vi "Database.Main-Select.vi"(8 "error in":errorcluster, 10 "Values":T1 {"Values" format="%.3f"}) -> (0 "error out":errorcluster, 2 "Saved":bool)   [LabVIEW 2016]
doc: "Go to DB->WriteStationValues action\nReturn boolean flag to show if data was saved to DB successfully\n\nWabco 2017 All right reserved\nAuthor: maciej.szupienko@wabco-auto.com"
uses:
  Database.Main.Data.PrevStation.ctl
  Sequence/Sequence.Step.Status.ctl
  Database.Main.Action.ctl
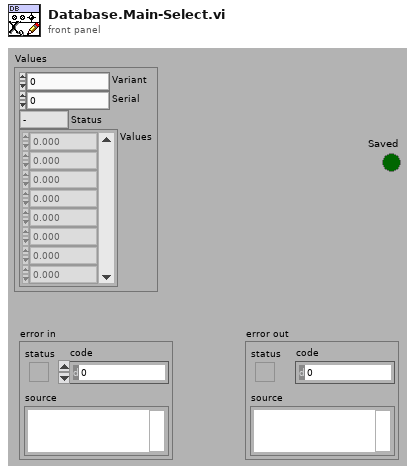
[diagram p1: front panel]
types:
  T1 = typedef "Database.Main.Data.PrevStation.ctl" = cluster{"Variant":u64, "Serial":u64, "Status":T2, "Values":dbl[]}
  T2 = typedef "Sequence.Step.Status.ctl" = enum16{"-", "Pending", "Running", "Skipped", "Passed", "Failed", "Done", "Error", "Aborted", "Stopped"}
  T3 = typedef "Database.Main.Action.ctl" = enum32{"idle", "constructor", "destructor", "--- DB ---", "Init", "Setup", "WriteStationValues"}
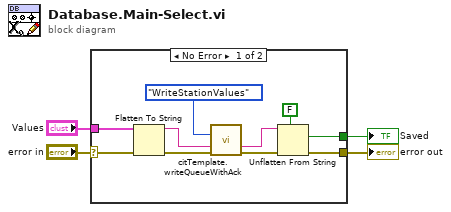
[diagram p0: block diagram]
diagram:
  n1 = case shown="No Error" "error in" {
    selector: "error in" -> [w14 w15]
    tunnel: [w9 w15] -> w3
    tunnel: "Values" -> [w13 _]
    tunnel: [w5 _] -> w1
    frame No Error {
      n2 = Flatten To String(anything=w13, error in (no error)=w14) -> (data string=w11:string, error out=w12:errorcluster)  [unwired: 2 in, 1 out]
      n3 = call "citTemplate.writeQueueWithAck.vi"("event in"=Database.Main.Action."WriteStationValues" ("Action"), "(flatten) data in"=w11, "error in (no error)"=w12) -> ("notification data"=w8:string, "error out"=w10:errorcluster)  [unwired: 10 in, 1 out]
      n4 = Unflatten From String(type=FALSE, binary string=w8, error in (no error)=w10) -> (value=w5:bool, error out=w9:errorcluster)  [unwired: 2 in, 1 out]
    }
    frame Error {
    }
  }
  "error out" <- w3
  "Saved" <- w1
